vi "AquaLogic_Test_Stand_v2.vi"() -> ()   [LabVIEW 2011]
panel:
  out "Save":T1={"Save Enable"=FALSE, "Save Interval [s]"=30.0, "Folder Location"=path "", "File Name"=""}
  in  "Save Interval [s]":dbl=30.0 min=0.0
  in  "Save Enable":bool
  in  "STOP PROGRAM":bool
  in  "MAIN TAB":T2(tab)=enum."PROGRAM CONFIG"
  in  "Display A":T3={"ON-DEMAND Display"=[{"CMD_Display"="User Parameter : 27 CURRCELL PWM Ramp", "Parameter Table"=[["Ramp Up Rate", "Ramp Down Rate", ""], ["0.000", "0.000", ""]], "SET"=FALSE, "GET"=FALSE}, {"CMD_Display"="User Parameter : 28 OUTPUT PWM Ramp", "Parameter Table"=[["Ramp Up Rate", "Ramp Down Rate", ""], ["0.000", "0.000", ""]], "SET"=FALSE, "GET"=FALSE}, {"CMD_Display"="User Parameter : 29 Cell Current SP / Status", "Parameter Table"=[["CURRCELL SP (amps)", "", ""], ["0.000", "", ""]], "SET"=FALSE, "GET"=FALSE}], "CONTINUOUS Display"=[{"CMD_Display"="DU:41  Temperature Measurements", "Param Output"=[["PCB Temperature (°F)", "External Temp (°F)", "Cond Temp (°F)"], ["PCB Temperature (°F)", "External Temp (°F)", "Cond Temp (°F)"]]}], "ERROR List"=[], "STATUS List"=[], "DIGITAL List"=[], "ERROR_SCROLL"=0, "STATUS_SCROLL"=0, "DIGITAL_SCROLL"=0}
  in  "Display B":T3={"ON-DEMAND Display"=[{"CMD_Display"="User Parameter : 20 Conductivity Thresholds", "Parameter Table"=[[">= Water Presence", ">= Low Salt", "<= Out of Salt [OFF]"], ["08.000", "10.000", "12.000"]], "SET"=FALSE, "GET"=FALSE}, {"CMD_Display"="User Parameter : 22 PCB Temp Threshold", "Parameter Table"=[[">= Max PCB Temp (°F)", "", ""], ["200.00", "", ""]], "SET"=FALSE, "GET"=FALSE}, {"CMD_Display"="User Parameter : 24 DayTank Setpoints", "Parameter Table"=[["<= Min / Empty Tank", ">= Fill Setpoint", ">= Tank Overfill"], ["00.500", "00.750", "01.250"]], "SET"=FALSE, "GET"=FALSE}, {"CMD_Display"="User Parameter : 25 Voltage Thresholds", "Parameter Table"=[["<= Min / Failure", ">= Low Salt", ">= Max / Failure"], ["00.000", "15.000", "20.000"]], "SET"=FALSE, "GET"=FALSE}, {"CMD_Display"="User Parameter : 26 Current Setpoint Limits", "Parameter Table"=[["Minimum Current (amps)", "Maximum Current (amps)", ""], ["00.000", "15.000", ""]], "SET"=FALSE, "GET"=FALSE}, {"CMD_Display"="User Parameter : 27 CURRCELL PWM Ramp", "Parameter Table"=[["Ramp Up Rate", "Ramp Down Rate", ""], ["00.250", "15.000", ""]], "SET"=FALSE, "GET"=FALSE}, {"CMD_Display"="User Parameter : 28 OUTPUT PWM Ramp", "Parameter Table"=[["Ramp Up Rate", "Ramp Down Rate", ""], ["00.500", "01.000", ""]], "SET"=FALSE, "GET"=FALSE}, {"CMD_Display"="User Parameter : 29 Cell Current SP / Status", "Parameter Table"=[["CURRCELL SP (amps)", "", ""], ["00.000", "", ""]], "SET"=FALSE, "GET"=FALSE}, {"CMD_Display"="User Parameter : 30 PWM Output 1 Setpoint", "Parameter Table"=[["Duty Cycle SP (%)", "", ""], ["0.00", "", ""]], "SET"=FALSE, "GET"=FALSE}, {"CMD_Display"="User Parameter : 31 PWM Output 2 Setpoint", "Parameter Table"=[["Duty Cycle SP (%)", "", ""], ["000.00", "", ""]], "SET"=FALSE, "GET"=FALSE}, {"CMD_Display"="User Parameter : 32 PWM Output 3 Setpoint", "Parameter Table"=[["Duty Cycle SP (%)", "", ""], ["000.00", "", ""]], "SET"=FALSE, "GET"=FALSE}], "CONTINUOUS Display"=[{"CMD_Display"="DU:33  Cell Status", "Param Output"=[["CELLDRIVE Duty (%)", "VOLTSCELL (volts)", "CURRCELL (amps)"], ["000.00", "00.000", "00.015"]]}, {"CMD_Display"="DU:34  PWM1 Status", "Param Output"=[["Duty Cycle (%)", "EMFOUT (volts)", "OVRCOUT (amps)"], ["000.00", "00.765", "00.000"]]}, {"CMD_Display"="DU:41  Temperature Measurements", "Param Output"=[["PCB Temperature (°F)", "Conductivity Temp (°F)", ""], ["069.91", "Conductivity Temp (°F)", ""]]}], "ERROR List"=[], "STATUS List"=[], "DIGITAL List"=[], "ERROR_SCROLL"=0, "STATUS_SCROLL"=0, "DIGITAL_SCROLL"=0}
  in  "Display C":T3={"ON-DEMAND Display"=[{"CMD_Display"="User Parameter : 20 Conductivity Thresholds", "Parameter Table"=[[">= Water Presence", ">= Low Salt", "<= Out of Salt [OFF]"], ["08.000", "10.000", "12.000"]], "SET"=FALSE, "GET"=FALSE}, {"CMD_Display"="User Parameter : 22 PCB Temp Threshold", "Parameter Table"=[[">= Max PCB Temp (°F)", "", ""], ["200.00", "", ""]], "SET"=FALSE, "GET"=FALSE}, {"CMD_Display"="User Parameter : 24 DayTank Setpoints", "Parameter Table"=[["<= Min / Empty Tank", ">= Fill Setpoint", ">= Tank Overfill"], ["00.500", "00.750", "01.250"]], "SET"=FALSE, "GET"=FALSE}, {"CMD_Display"="User Parameter : 25 Voltage Thresholds", "Parameter Table"=[["<= Min / Failure", ">= Low Salt", ">= Max / Failure"], ["00.000", "15.000", "20.000"]], "SET"=FALSE, "GET"=FALSE}, {"CMD_Display"="User Parameter : 26 Current Setpoint Limits", "Parameter Table"=[["Minimum Current (amps)", "Maximum Current (amps)", ""], ["00.000", "15.000", ""]], "SET"=FALSE, "GET"=FALSE}, {"CMD_Display"="User Parameter : 27 CURRCELL PWM Ramp", "Parameter Table"=[["Ramp Up Rate", "Ramp Down Rate", ""], ["00.250", "15.000", ""]], "SET"=FALSE, "GET"=FALSE}, {"CMD_Display"="User Parameter : 28 OUTPUT PWM Ramp", "Parameter Table"=[["Ramp Up Rate", "Ramp Down Rate", ""], ["00.500", "01.000", ""]], "SET"=FALSE, "GET"=FALSE}, {"CMD_Display"="User Parameter : 29 Cell Current SP / Status", "Parameter Table"=[["CURRCELL SP (amps)", "", ""], ["00.000", "", ""]], "SET"=FALSE, "GET"=FALSE}, {"CMD_Display"="User Parameter : 30 PWM Output 1 Setpoint", "Parameter Table"=[["Duty Cycle SP (%)", "", ""], ["0.00", "", ""]], "SET"=FALSE, "GET"=FALSE}, {"CMD_Display"="User Parameter : 31 PWM Output 2 Setpoint", "Parameter Table"=[["Duty Cycle SP (%)", "", ""], ["000.00", "", ""]], "SET"=FALSE, "GET"=FALSE}, {"CMD_Display"="User Parameter : 32 PWM Output 3 Setpoint", "Parameter Table"=[["Duty Cycle SP (%)", "", ""], ["000.00", "", ""]], "SET"=FALSE, "GET"=FALSE}], "CONTINUOUS Display"=[{"CMD_Display"="DU:33  Cell Status", "Param Output"=[["CELLDRIVE Duty (%)", "VOLTSCELL (volts)", "CURRCELL (amps)"], ["000.00", "00.000", "00.015"]]}, {"CMD_Display"="DU:34  PWM1 Status", "Param Output"=[["Duty Cycle (%)", "EMFOUT (volts)", "OVRCOUT (amps)"], ["000.00", "00.765", "00.000"]]}, {"CMD_Display"="DU:41  Temperature Measurements", "Param Output"=[["PCB Temperature (°F)", "Conductivity Temp (°F)", ""], ["069.91", "Conductivity Temp (°F)", ""]]}], "ERROR List"=[], "STATUS List"=[], "DIGITAL List"=[], "ERROR_SCROLL"=0, "STATUS_SCROLL"=0, "DIGITAL_SCROLL"=0}
  in  "Display D":T3={"ON-DEMAND Display"=[{"CMD_Display"="User Parameter : 20 Conductivity Thresholds", "Parameter Table"=[[">= Water Presence", ">= Low Salt", "<= Out of Salt [OFF]"], ["08.000", "10.000", "12.000"]], "SET"=FALSE, "GET"=FALSE}, {"CMD_Display"="User Parameter : 22 PCB Temp Threshold", "Parameter Table"=[[">= Max PCB Temp (°F)", "", ""], ["200.00", "", ""]], "SET"=FALSE, "GET"=FALSE}, {"CMD_Display"="User Parameter : 24 DayTank Setpoints", "Parameter Table"=[["<= Min / Empty Tank", ">= Fill Setpoint", ">= Tank Overfill"], ["00.500", "00.750", "01.250"]], "SET"=FALSE, "GET"=FALSE}, {"CMD_Display"="User Parameter : 25 Voltage Thresholds", "Parameter Table"=[["<= Min / Failure", ">= Low Salt", ">= Max / Failure"], ["00.000", "15.000", "20.000"]], "SET"=FALSE, "GET"=FALSE}, {"CMD_Display"="User Parameter : 26 Current Setpoint Limits", "Parameter Table"=[["Minimum Current (amps)", "Maximum Current (amps)", ""], ["00.000", "15.000", ""]], "SET"=FALSE, "GET"=FALSE}, {"CMD_Display"="User Parameter : 27 CURRCELL PWM Ramp", "Parameter Table"=[["Ramp Up Rate", "Ramp Down Rate", ""], ["00.250", "15.000", ""]], "SET"=FALSE, "GET"=FALSE}, {"CMD_Display"="User Parameter : 28 OUTPUT PWM Ramp", "Parameter Table"=[["Ramp Up Rate", "Ramp Down Rate", ""], ["00.500", "01.000", ""]], "SET"=FALSE, "GET"=FALSE}, {"CMD_Display"="User Parameter : 29 Cell Current SP / Status", "Parameter Table"=[["CURRCELL SP (amps)", "", ""], ["00.000", "", ""]], "SET"=FALSE, "GET"=FALSE}, {"CMD_Display"="User Parameter : 30 PWM Output 1 Setpoint", "Parameter Table"=[["Duty Cycle SP (%)", "", ""], ["0.00", "", ""]], "SET"=FALSE, "GET"=FALSE}, {"CMD_Display"="User Parameter : 31 PWM Output 2 Setpoint", "Parameter Table"=[["Duty Cycle SP (%)", "", ""], ["000.00", "", ""]], "SET"=FALSE, "GET"=FALSE}, {"CMD_Display"="User Parameter : 32 PWM Output 3 Setpoint", "Parameter Table"=[["Duty Cycle SP (%)", "", ""], ["000.00", "", ""]], "SET"=FALSE, "GET"=FALSE}], "CONTINUOUS Display"=[{"CMD_Display"="DU:33  Cell Status", "Param Output"=[["CELLDRIVE Duty (%)", "VOLTSCELL (volts)", "CURRCELL (amps)"], ["000.00", "00.000", "00.015"]]}, {"CMD_Display"="DU:34  PWM1 Status", "Param Output"=[["Duty Cycle (%)", "EMFOUT (volts)", "OVRCOUT (amps)"], ["000.00", "00.765", "00.000"]]}, {"CMD_Display"="DU:41  Temperature Measurements", "Param Output"=[["PCB Temperature (°F)", "Conductivity Temp (°F)", ""], ["069.91", "Conductivity Temp (°F)", ""]]}], "ERROR List"=[], "STATUS List"=[], "DIGITAL List"=[], "ERROR_SCROLL"=0, "STATUS_SCROLL"=0, "DIGITAL_SCROLL"=0}
  in  "ESP Table Cluster":T4={"ON-DEMAND Config"=FALSE, "ON-DEMAND Active Commands"=[27, 28, 29], "CONTINUOUS Config"=FALSE, "CONTINUOUS Active Commands"=[41], "ERROR Config"=FALSE, "ERROR Command"="38", "STATUS Config"=FALSE, "STATUS Command"="37", "DIGITAL Config"=FALSE, "DIGITAL Command"="39", "SAVE TABLE"=FALSE, "Active Table"=0, "New Table Name"="7-16-2012 new", "NEW CMD TABLE"=[22]} {"Active Table" items=["No Tables Found"]}
  in  "Config Sub-Tab":T5(tab)=enum."General"
  out "ESP Error A":errorcluster
  out "ESP Output A":T6={"Write Command"="\u0001eb:DU:38:A600\u0004", "Read String"="", "Read Bytes"=0, "Bytes at Port"=0, "Response"="", "ACK"=FALSE, "EOT"=FALSE, "NAK"=FALSE, "Parameters"=[]}
  in  "ESP Config A":T7={"COM Port Input"="COM1", "Manual Command"={"Device Type"="", "Instance"="", "Command"="", "Sub-Command"="", "Parameters (Seperate by :)"=""}, "Device Type"="e", "Instance"="a", "Use Manual Command?"=FALSE, "Timeout [msec]"=1000, "Read/Write Wait [msec]"=25}
  out "ESP Error B":errorcluster
  out "ESP Output B":T6={"Write Command"="\u0001eb:DU:38:A600\u0004", "Read String"="", "Read Bytes"=0, "Bytes at Port"=0, "Response"="", "ACK"=FALSE, "EOT"=FALSE, "NAK"=FALSE, "Parameters"=[]}
  in  "ESP Config B":T7={"COM Port Input"="COM1", "Manual Command"={"Device Type"="", "Instance"="", "Command"="", "Sub-Command"="", "Parameters (Seperate by :)"=""}, "Device Type"="e", "Instance"="b", "Use Manual Command?"=FALSE, "Timeout [msec]"=1000, "Read/Write Wait [msec]"=25}
  out "ESP Error C":errorcluster
  out "ESP Output C":T6={"Write Command"="\u0001eb:DU:38:A600\u0004", "Read String"="", "Read Bytes"=0, "Bytes at Port"=0, "Response"="", "ACK"=FALSE, "EOT"=FALSE, "NAK"=FALSE, "Parameters"=[]}
  in  "ESP Config C":T7={"COM Port Input"="COM2", "Manual Command"={"Device Type"="", "Instance"="", "Command"="", "Sub-Command"="", "Parameters (Seperate by :)"=""}, "Device Type"="e", "Instance"="a", "Use Manual Command?"=FALSE, "Timeout [msec]"=1000, "Read/Write Wait [msec]"=25}
  out "ESP Error D":errorcluster
  out "ESP Output D":T6={"Write Command"="\u0001eb:DU:38:A600\u0004", "Read String"="", "Read Bytes"=0, "Bytes at Port"=0, "Response"="", "ACK"=FALSE, "EOT"=FALSE, "NAK"=FALSE, "Parameters"=[]}
  in  "ESP Config D":T7={"COM Port Input"="COM2", "Manual Command"={"Device Type"="", "Instance"="", "Command"="", "Sub-Command"="", "Parameters (Seperate by :)"=""}, "Device Type"="e", "Instance"="b", "Use Manual Command?"=FALSE, "Timeout [msec]"=1000, "Read/Write Wait [msec]"=25}
  in  "Table Location":path
  in  "Save Location":path
  in  "File Name":string
  out "Numeric":i32=32
  in  "Loop Wait [ms] B":u32=1
  out "Loop Time [ms] B":u32=1
  in  "Loop Wait [ms] C":u32=1
  out "Loop Time [ms] C":u32=1
  out "Loop Time [ms] D":u32=1
  in  "Loop Wait [ms] A":u32=1
  in  "Loop Wait [ms] D":u32=1
  out "Loop Time [ms] A":u32=1
  in  "Enable B":bool
  in  "Enable A":bool
  in  "Enable C":bool
  in  "Enable D":bool
  out "Table Error":errorcluster
  out "SYSTEM OK":bool
  # "AQUALOGIC \nLabVIEW Test Interface"
  # "Blake Otting - 2012"
  # "On-Demand ESP Commands (DU and SU)"
  # "Continuous-Read ESP Commands (DU)"
  # "On-Demand ESP Commands (DU and SU)"
  # "Continuous-Read ESP Commands (DU)"
  # "On-Demand ESP Commands (DU and SU)"
  # "Continuous-Read ESP Commands (DU)"
  # "On-Demand ESP Commands (DU and SU)"
  # "Continuous-Read ESP Commands (DU)"
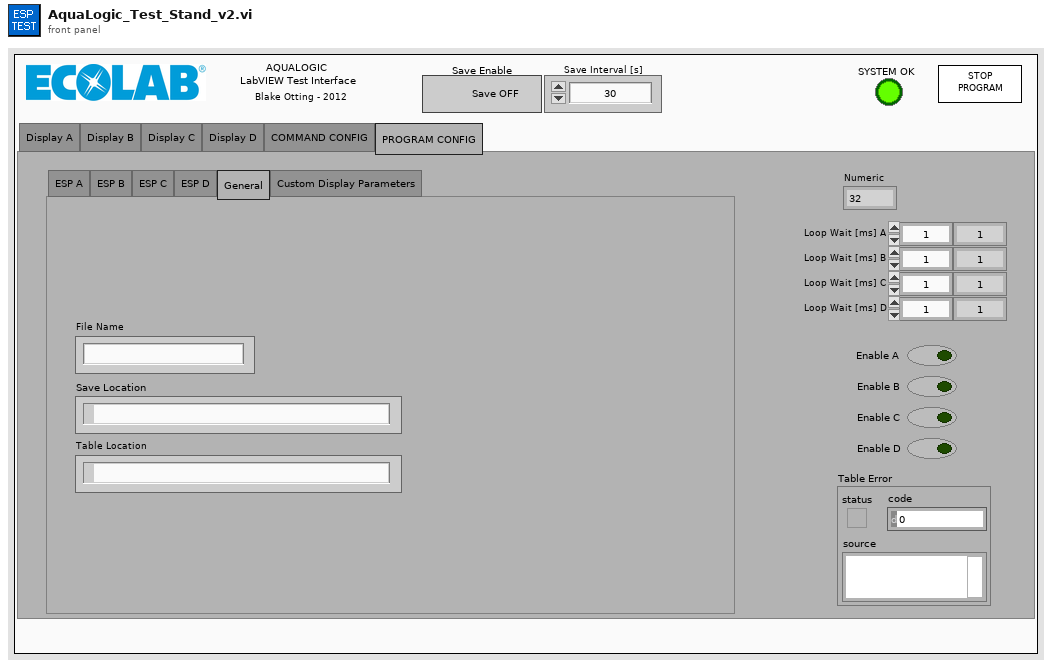
[diagram p1: front panel]
types:
  T1 = cluster{"Save Enable":bool, "Save Interval [s]":dbl, "Folder Location":path, "File Name":string}
  T2 = enum32{"Display A", "Display B", "Display C", "Display D", "COMMAND CONFIG", "PROGRAM CONFIG"}
  T3 = cluster{"ON-DEMAND Display":cluster{"CMD_Display":string, "Parameter Table":string[][], "SET":bool, "GET":bool}[], "CONTINUOUS Display":cluster{"CMD_Display":string, "Param Output":string[][]}[], "ERROR List":i32[], "STATUS List":i32[], "DIGITAL List":i32[], "ERROR_SCROLL":u8, "STATUS_SCROLL":u8, "DIGITAL_SCROLL":u8}
  T4 = cluster{"ON-DEMAND Config":bool, "ON-DEMAND Active Commands":i32[], "CONTINUOUS Config":bool, "CONTINUOUS Active Commands":i32[], "ERROR Config":bool, "ERROR Command":string, "STATUS Config":bool, "STATUS Command":string, "DIGITAL Config":bool, "DIGITAL Command":string, "SAVE TABLE":bool, "Active Table":u16, "New Table Name":string, "NEW CMD TABLE":i32[]}
  T5 = enum32{"ESP A", "ESP B", "ESP C", "ESP D", "General", "Custom Display Parameters"}
  T6 = cluster{"Write Command":string, "Read String":string, "Read Bytes":u32, "Bytes at Port":u32, "Response":string, "ACK":bool, "EOT":bool, "NAK":bool, "Parameters":string[]}
  T7 = cluster{"COM Port Input":refnum<visa-resource-name>, "Manual Command":cluster{"Device Type":string, "Instance":string, "Command":string, "Sub-Command":string, "Parameters (Seperate by :)":string}, "Device Type":string, "Instance":string, "Use Manual Command?":bool, "Timeout [msec]":u32, "Read/Write Wait [msec]":u32}
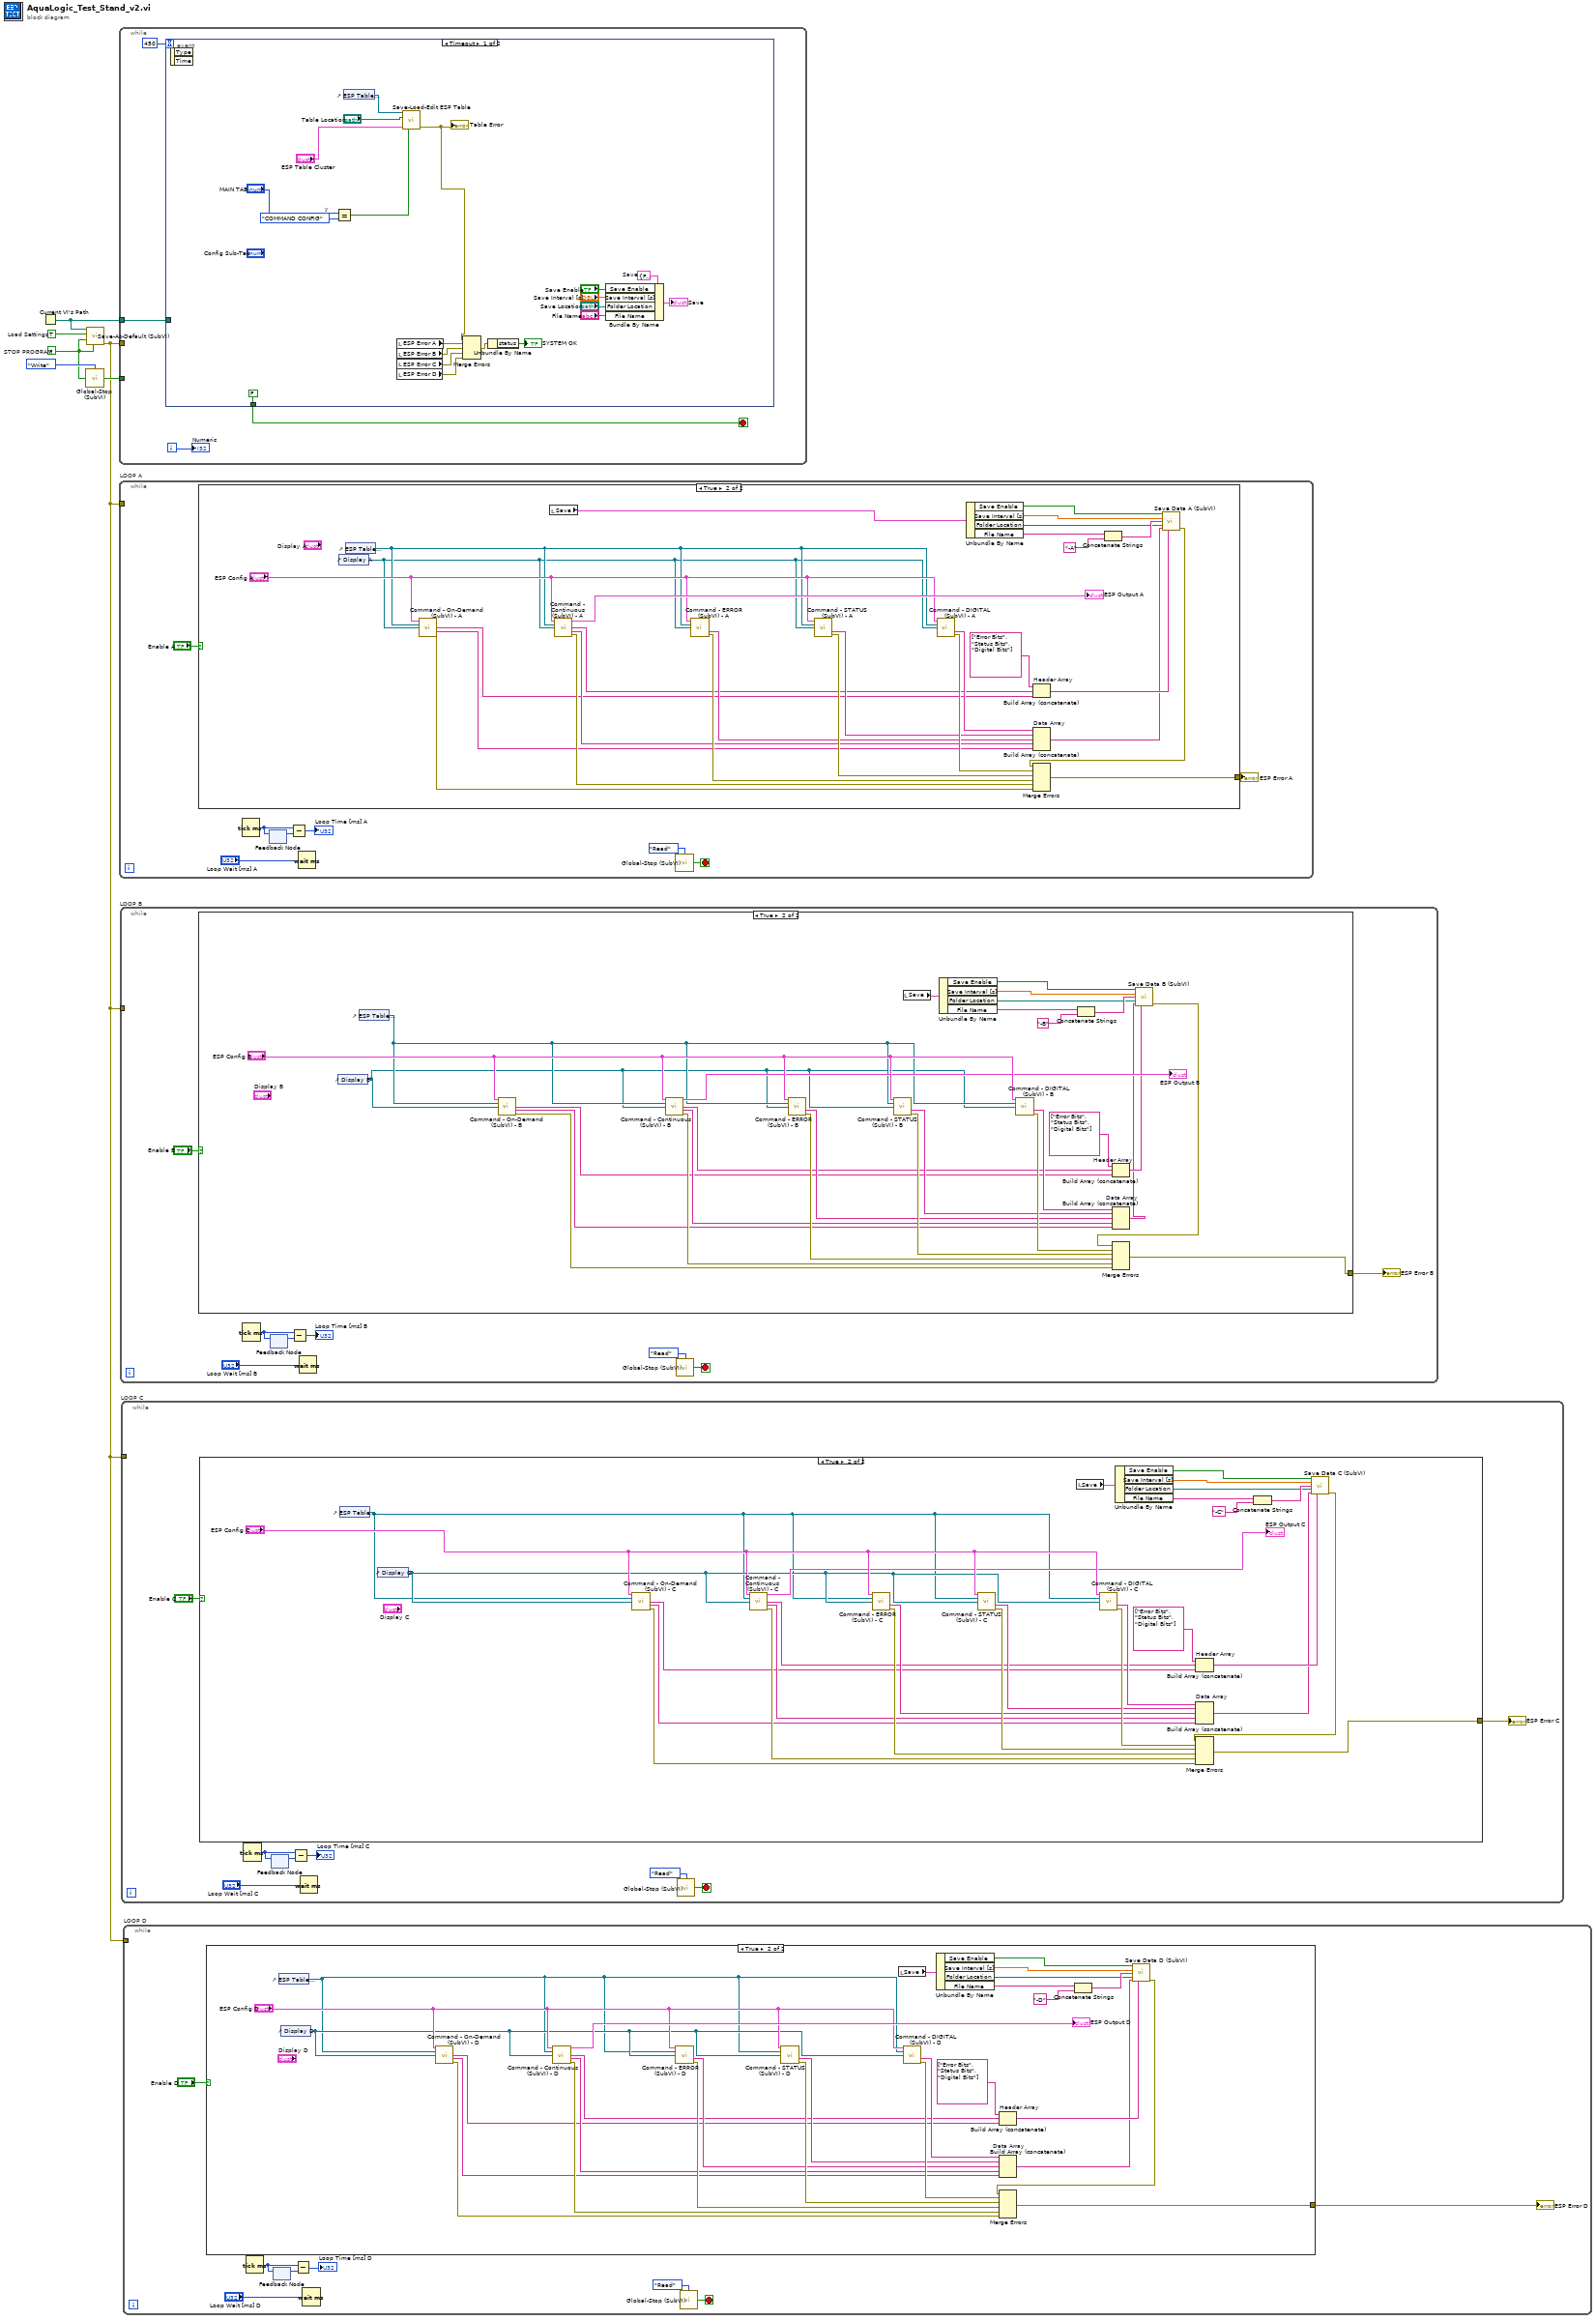
[diagram p0: block diagram]
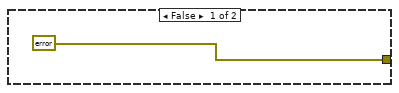
[diagram p2: hidden frame]
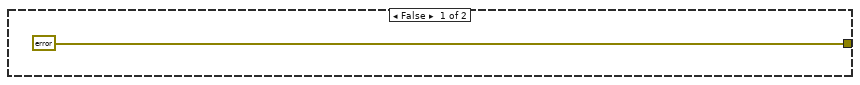
[diagram p3: hidden frame]
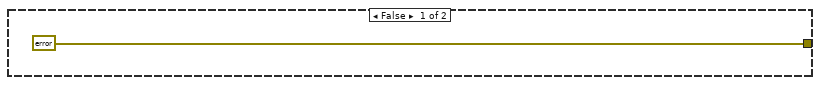
[diagram p4: hidden frame]
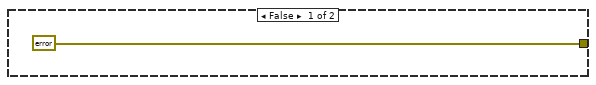
[diagram p5: hidden frame]
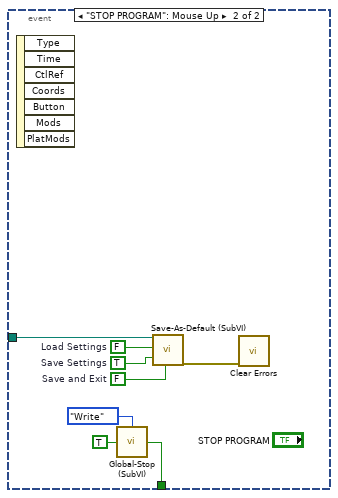
[diagram p6: hidden frame]
diagram:
  w6 = TRUE  # Load Settings
  w2 = FALSE  # STOP PROGRAM
  n1 = Current VI's Path() -> (path=w3:path)
  n2 = call "Global-Stop (SubVI).vi"("Mode (Read)"=enum16{"Read", "Write"}."Write", "IN"=w2) -> ("OUT"=w4:bool)  [unwired: 2 in]
  n3 = call "Save-As-Default (SubVI).vi"("Current VI's Path"=w3, "Load Settings"=w6, "Save Settings"=w2, "Save and Exit"=w2) -> ("Save as Default Error"=w1:errorcluster)  [unwired: 15 in]
  n4 = while {
    tunnel: w4 -> [_]
    tunnel: w3 -> [w7]
    tunnel: w1 -> [_]
    i -> [w8]
    stop <- w10 stop-if-true
    n5 = event shown="[0] Timeout" {
      selector: _ -> [_ _]
      dyn-events: _ -> [_ _]
      timeout: 450 -> [_ _]
      tunnel: [FALSE w38] -> w10
      tunnel: w7 -> [_ w31]
      event Timeout {
        w14 = T2."COMMAND CONFIG"  # y
        w30 = T1 {"Save Enable"=FALSE, "Save Interval [s]"=30.0, "Folder Location"=path "", "File Name"=""}  # Save
        n6 = event-data() -> ()  [unwired: 1 in, 2 out]
        n7 = Equal?(x="MAIN TAB", y=w14) -> (x = y?=w12:bool)
        n8 = control-ref of="ESP Table Cluster"() -> (w13:refnum<vi>)
        n9 = local read "ESP Error A"() -> (w23:errorcluster)
        n10 = local read "ESP Error B"() -> (w20:errorcluster)
        n11 = local read "ESP Error C"() -> (w19:errorcluster)
        n12 = local read "ESP Error D"() -> (w18:errorcluster)
        n13 = call "Save-Load-Edit ESP Table.vi"(0:"ESP Table Cluster"=w13, "Table Folder"="Table Location", 11:"ESP Table Cluster"="ESP Table Cluster", "ENABLE"=w12) -> ("Error Output"=w16:errorcluster)  [unwired: 11 in]
        "Table Error" <- w16
        n14 = Merge Errors(w16, w23, w20, w19, w18) -> (w22:errorcluster)
        n15 = Unbundle By Name(w22) -> ("status"=→"SYSTEM OK":bool)
        n16 = Bundle By Name(cluster=w30, "Save Enable"="Save Enable", "Save Interval [s]"="Save Interval [s]", "Folder Location"="Save Location", "File Name"="File Name") -> (→"Save":T1)
      }
      event "STOP PROGRAM": Mouse Up {
        w33 = FALSE  # Save and Exit
        w34 = TRUE  # Save Settings
        w35 = FALSE  # Load Settings
        n17 = event-data() -> ()  [unwired: 1 in, 7 out]
        n18 = call "Global-Stop (SubVI).vi"("Mode (Read)"=enum16{"Read", "Write"}."Write", "IN"=TRUE) -> ("OUT"=w38:bool)  [unwired: 2 in]
        n19 = call "Save-As-Default (SubVI).vi"("Current VI's Path"=w31, "Load Settings"=w35, "Save Settings"=w34, "Save and Exit"=w33) -> ("Save as Default Error"=w32:errorcluster)  [unwired: 15 in]
        n20 = call <vilib>:"Clear Errors.vi"("error in (no error)"=w32) -> ()  [unwired: 6 in, 1 out]
      }
    }
    "Numeric" <- w8
  }
  n21 = while "LOOP A" {
    tunnel: w1 -> [_]
    stop <- w45 stop-if-true
    n22 = case shown="True" "Enable A" {
      tunnel: [errorcluster {"status"=FALSE, "code"=0, "source"=""} w69] -> w40
      frame False {
      }
      frame True {
        n23 = control-ref of="Display A"() -> (w48:refnum<vi>)
        n24 = control-ref of="ESP Table Cluster"() -> (w49:refnum<vi>)
        n25 = call "Command - On-Demand (SubVI) - A.vi"("ESP Config"="ESP Config A", "ESP Table Cluster Ref"=w49, "Display Cluster Ref"=w48) -> ("On-Demand Header"=w53:string[], "On-Demand Data"=w59:string[], "ON Demand"=w64:errorcluster)  [unwired: 9 in, 1 out]
        n26 = local read "Save"() -> (w68:T1)
        n27 = call "Command - Continuous (SubVI) - A.vi"("ESP Config"="ESP Config A", "ESP Table Cluster Ref"=w49, "Display Cluster Ref"=w48) -> ("ESP Values"=→"ESP Output A":T6, "Continuous Header"=w54:string[], "Continuous Data"=w58:string[], "CONTINUOUS ERR"=w63:errorcluster)  [unwired: 8 in, 1 out]
        n28 = call "Command - ERROR (SubVI) - A.vi"("ESP Config"="ESP Config A", "ESP Table Cluster Ref"=w49, "Display Cluster Ref"=w48) -> ("ERROR Data"=w57:string, "ERROR List"=w62:errorcluster)  [unwired: 11 in]
        n29 = call "Command - STATUS (SubVI) - A.vi"("ESP Config"="ESP Config A", "ESP Table Cluster Ref"=w49, "Display Cluster Ref"=w48) -> ("STATUS Data"=w56:string, "STATUS List"=w61:errorcluster)  [unwired: 11 in]
        n30 = call "Command - DIGITAL (SubVI) - A.vi"("ESP Config"="ESP Config A", "ESP Table Cluster Ref"=w49, "Display Cluster Ref"=w48) -> ("DIGITAL Data"=w55:string, "DIGITAL List"=w60:errorcluster)  [unwired: 11 in]
        n31 = Unbundle By Name(w68) -> ("Save Enable"=w70:bool, "Save Interval [s]"=w71:dbl, "Folder Location"=w72:path, "File Name"=w73:string)
        n32 = Build Array (concatenate) "Header Array"(string[] ["Error Bits", "Status Bits", "Digital Bits"], w54, w53) -> (w52:string[])
        n33 = Build Array (concatenate) "Data Array"(w55, w56, w57, w58, w59) -> (w51:string[])
        n34 = Concatenate Strings(w73, "-A") -> (w74:string)
        n35 = call "Save Data A (SubVI).vi"("Save Enable"=w70, "Save Interval [s]"=w71, "File Name"=w74, "Folder Location"=w72, "Data Array (Row)"=w51, "Column Header Array"=w52) -> ("Save Error"=w50:errorcluster)  [unwired: 7 in, 2 out]
        n36 = Merge Errors(w50, w60, w61, w62, w63, w64) -> (w69:errorcluster)
      }
    }
    "ESP Error A" <- w40
    n37 = Tick Count (ms)() -> (millisecond timer value=w43:u32)
    n38 = feedback #1() -> (w42:u32)  [unwired: 1 in]
    n39 = feedback-in #1(w43) -> ()
    n40 = Subtract(x=w43, y=w42) -> (x-y=→"Loop Time [ms] A":u32)
    n41 = Wait (ms)(milliseconds to wait="Loop Wait [ms] A") -> ()  [unwired: 1 out]
    n42 = call "Global-Stop (SubVI).vi"("Mode (Read)"=enum16{"Read", "Write"}."Read") -> ("OUT"=w45:bool)  [unwired: 3 in]
  }
  n43 = while "LOOP B" {
    tunnel: w1 -> [_]
    stop <- w82 stop-if-true
    n44 = case shown="True" "Enable B" {
      tunnel: [errorcluster {"status"=FALSE, "code"=0, "source"=""} w87] -> w76
      frame False {
      }
      frame True {
        n45 = control-ref of="Display B"() -> (w85:refnum<vi>)
        n46 = control-ref of="ESP Table Cluster"() -> (w86:refnum<vi>)
        n47 = call "Command - On-Demand (SubVI) - B.vi"("ESP Config"="ESP Config B", "ESP Table Cluster Ref"=w86, "Display Cluster Ref"=w85) -> ("On-Demand Header"=w90:string[], "On-Demand Data"=w96:string[], "ON Demand"=w101:errorcluster)  [unwired: 9 in, 1 out]
        n48 = call "Command - Continuous (SubVI) - B.vi"("ESP Config"="ESP Config B", "ESP Table Cluster Ref"=w86, "Display Cluster Ref"=w85) -> ("ESP Values"=→"ESP Output B":T6, "Continuous Header"=w91:string[], "Continuous Data"=w95:string[], "CONTINUOUS ERR"=w100:errorcluster)  [unwired: 8 in, 1 out]
        n49 = call "Command - ERROR (SubVI) - B.vi"("ESP Config"="ESP Config B", "ESP Table Cluster Ref"=w86, "Display Cluster Ref"=w85) -> ("ERROR Data"=w94:string, "ERROR List"=w99:errorcluster)  [unwired: 11 in]
        n50 = call "Command - STATUS (SubVI) - B.vi"("ESP Config"="ESP Config B", "ESP Table Cluster Ref"=w86, "Display Cluster Ref"=w85) -> ("STATUS Data"=w93:string, "STATUS List"=w98:errorcluster)  [unwired: 11 in]
        n51 = local read "Save"() -> (w103:T1)
        n52 = Unbundle By Name(w103) -> ("Save Enable"=w107:bool, "Save Interval [s]"=w108:dbl, "Folder Location"=w109:path, "File Name"=w110:string)
        n53 = call "Command - DIGITAL (SubVI) - B.vi"("ESP Config"="ESP Config B", "ESP Table Cluster Ref"=w86, "Display Cluster Ref"=w85) -> ("DIGITAL Data"=w92:string, "DIGITAL List"=w97:errorcluster)  [unwired: 11 in]
        n54 = Concatenate Strings(w110, "-B") -> (w111:string)
        n55 = Build Array (concatenate) "Header Array"(string[] ["Error Bits", "Status Bits", "Digital Bits"], w91, w90) -> (w89:string[])
        n56 = Build Array (concatenate) "Data Array"(w92, w93, w94, w95, w96) -> (w88:string[])
        n57 = call "Save Data B (SubVI).vi"("Save Enable"=w107, "Save Interval [s]"=w108, "File Name"=w111, "Folder Location"=w109, "Data Array (Row)"=w88, "Column Header Array"=w89) -> ("Save Error"=w105:errorcluster)  [unwired: 7 in, 2 out]
        n58 = Merge Errors(w105, w97, w98, w99, w100, w101) -> (w87:errorcluster)
      }
    }
    "ESP Error B" <- w76
    n59 = Tick Count (ms)() -> (millisecond timer value=w80:u32)
    n60 = feedback #2() -> (w79:u32)  [unwired: 1 in]
    n61 = feedback-in #2(w80) -> ()
    n62 = Subtract(x=w80, y=w79) -> (x-y=→"Loop Time [ms] B":u32)
    n63 = Wait (ms)(milliseconds to wait="Loop Wait [ms] B") -> ()  [unwired: 1 out]
    n64 = call "Global-Stop (SubVI).vi"("Mode (Read)"=enum16{"Read", "Write"}."Read") -> ("OUT"=w82:bool)  [unwired: 3 in]
  }
  n65 = while "LOOP C" {
    tunnel: w1 -> [_]
    stop <- w119 stop-if-true
    n66 = case shown="True" "Enable C" {
      tunnel: [errorcluster {"status"=FALSE, "code"=0, "source"=""} w124] -> w113
      frame False {
      }
      frame True {
        n67 = control-ref of="ESP Table Cluster"() -> (w122:refnum<vi>)
        n68 = control-ref of="Display C"() -> (w123:refnum<vi>)
        n69 = call "Command - On-Demand (SubVI) - C.vi"("ESP Config"="ESP Config C", "ESP Table Cluster Ref"=w122, "Display Cluster Ref"=w123) -> ("On-Demand Header"=w126:string[], "On-Demand Data"=w132:string[], "ON Demand"=w137:errorcluster)  [unwired: 9 in, 1 out]
        n70 = call "Command - Continuous (SubVI) - C.vi"("ESP Config"="ESP Config C", "ESP Table Cluster Ref"=w122, "Display Cluster Ref"=w123) -> ("ESP Values"=→"ESP Output C":T6, "Continuous Header"=w127:string[], "Continuous Data"=w131:string[], "CONTINUOUS ERR"=w136:errorcluster)  [unwired: 8 in, 1 out]
        n71 = call "Command - ERROR (SubVI) - C.vi"("ESP Config"="ESP Config C", "ESP Table Cluster Ref"=w122, "Display Cluster Ref"=w123) -> ("ERROR Data"=w130:string, "ERROR List"=w135:errorcluster)  [unwired: 11 in]
        n72 = call "Command - STATUS (SubVI) - C.vi"("ESP Config"="ESP Config C", "ESP Table Cluster Ref"=w122, "Display Cluster Ref"=w123) -> ("STATUS Data"=w129:string, "STATUS List"=w134:errorcluster)  [unwired: 11 in]
        n73 = local read "Save"() -> (w142:T1)
        n74 = call "Command - DIGITAL (SubVI) - C.vi"("ESP Config"="ESP Config C", "ESP Table Cluster Ref"=w122, "Display Cluster Ref"=w123) -> ("DIGITAL Data"=w128:string, "DIGITAL List"=w133:errorcluster)  [unwired: 11 in]
        n75 = Unbundle By Name(w142) -> ("Save Enable"=w144:bool, "Save Interval [s]"=w145:dbl, "Folder Location"=w146:path, "File Name"=w147:string)
        n76 = Build Array (concatenate) "Header Array"(string[] ["Error Bits", "Status Bits", "Digital Bits"], w127, w126) -> (w140:string[])
        n77 = Build Array (concatenate) "Data Array"(w128, w129, w130, w131, w132) -> (w139:string[])
        n78 = Concatenate Strings(w147, "-C") -> (w148:string)
        n79 = call "Save Data C (SubVI).vi"("Save Enable"=w144, "Save Interval [s]"=w145, "File Name"=w148, "Folder Location"=w146, "Data Array (Row)"=w139, "Column Header Array"=w140) -> ("Save Error"=w125:errorcluster)  [unwired: 7 in, 2 out]
        n80 = Merge Errors(w125, w133, w134, w135, w136, w137) -> (w124:errorcluster)
      }
    }
    "ESP Error C" <- w113
    n81 = Tick Count (ms)() -> (millisecond timer value=w117:u32)
    n82 = feedback #3() -> (w116:u32)  [unwired: 1 in]
    n83 = feedback-in #3(w117) -> ()
    n84 = Subtract(x=w117, y=w116) -> (x-y=→"Loop Time [ms] C":u32)
    n85 = Wait (ms)(milliseconds to wait="Loop Wait [ms] C") -> ()  [unwired: 1 out]
    n86 = call "Global-Stop (SubVI).vi"("Mode (Read)"=enum16{"Read", "Write"}."Read") -> ("OUT"=w119:bool)  [unwired: 3 in]
  }
  n87 = while "LOOP D" {
    tunnel: w1 -> [_]
    stop <- w156 stop-if-true
    n88 = case shown="True" "Enable D" {
      tunnel: [errorcluster {"status"=FALSE, "code"=0, "source"=""} w162] -> w150
      frame False {
      }
      frame True {
        n89 = control-ref of="ESP Table Cluster"() -> (w159:refnum<vi>)
        n90 = control-ref of="Display D"() -> (w160:refnum<vi>)
        n91 = call "Command - On-Demand (SubVI) - D.vi"("ESP Config"="ESP Config D", "ESP Table Cluster Ref"=w159, "Display Cluster Ref"=w160) -> ("On-Demand Header"=w167:string[], "On-Demand Data"=w173:string[], "ON Demand"=w178:errorcluster)  [unwired: 9 in, 1 out]
        n92 = call "Command - Continuous (SubVI) - D.vi"("ESP Config"="ESP Config D", "ESP Table Cluster Ref"=w159, "Display Cluster Ref"=w160) -> ("ESP Values"=→"ESP Output D":T6, "Continuous Header"=w168:string[], "Continuous Data"=w172:string[], "CONTINUOUS ERR"=w177:errorcluster)  [unwired: 8 in, 1 out]
        n93 = call "Command - ERROR (SubVI) - D.vi"("ESP Config"="ESP Config D", "ESP Table Cluster Ref"=w159, "Display Cluster Ref"=w160) -> ("ERROR Data"=w171:string, "ERROR List"=w176:errorcluster)  [unwired: 11 in]
        n94 = call "Command - STATUS (SubVI) - D.vi"("ESP Config"="ESP Config D", "ESP Table Cluster Ref"=w159, "Display Cluster Ref"=w160) -> ("STATUS Data"=w170:string, "STATUS List"=w175:errorcluster)  [unwired: 11 in]
        n95 = local read "Save"() -> (w180:T1)
        n96 = call "Command - DIGITAL (SubVI) - D.vi"("ESP Config"="ESP Config D", "ESP Table Cluster Ref"=w159, "Display Cluster Ref"=w160) -> ("DIGITAL Data"=w169:string, "DIGITAL List"=w174:errorcluster)  [unwired: 11 in]
        n97 = Unbundle By Name(w180) -> ("Save Enable"=w181:bool, "Save Interval [s]"=w182:dbl, "Folder Location"=w183:path, "File Name"=w184:string)
        n98 = Build Array (concatenate) "Header Array"(string[] ["Error Bits", "Status Bits", "Digital Bits"], w168, w167) -> (w164:string[])
        n99 = Build Array (concatenate) "Data Array"(w169, w170, w171, w172, w173) -> (w163:string[])
        n100 = Concatenate Strings(w184, "-D") -> (w185:string)
        n101 = call "Save Data D (SubVI).vi"("Save Enable"=w181, "Save Interval [s]"=w182, "File Name"=w185, "Folder Location"=w183, "Data Array (Row)"=w163, "Column Header Array"=w164) -> ("Save Error"=w166:errorcluster)  [unwired: 7 in, 2 out]
        n102 = Merge Errors(w166, w174, w175, w176, w177, w178) -> (w162:errorcluster)
      }
    }
    "ESP Error D" <- w150
    n103 = Tick Count (ms)() -> (millisecond timer value=w154:u32)
    n104 = feedback #4() -> (w153:u32)  [unwired: 1 in]
    n105 = feedback-in #4(w154) -> ()
    n106 = Subtract(x=w154, y=w153) -> (x-y=→"Loop Time [ms] D":u32)
    n107 = Wait (ms)(milliseconds to wait="Loop Wait [ms] D") -> ()  [unwired: 1 out]
    n108 = call "Global-Stop (SubVI).vi"("Mode (Read)"=enum16{"Read", "Write"}."Read") -> ("OUT"=w156:bool)  [unwired: 3 in]
  }
